vi "CombineVIScreenshots.vi"(6 "Image Types":T1[](array[typedef]), 8 "error in (no error)":errorcluster, 9 "Output Folders":T5, 10 "VI 2 Screenshots in":T2, 11 "VI 1 Screenshots in":T2) -> (0 "error out":errorcluster)   [LabVIEW 2015, in "VIDiff_Screenshots.lvlib"]
uses:
  Screenshots/VIDiff_Screenshots.lvlib
  Utilities/Output Folders.ctl
  Screenshots/VI Screenshots.ctl
  Screenshots/Screenshot Info.ctl
  Screenshots/Screenshot Type.ctl
  Utilities/FilePaths.ctl
  Utilities/VIDiff_Utilities.lvlib
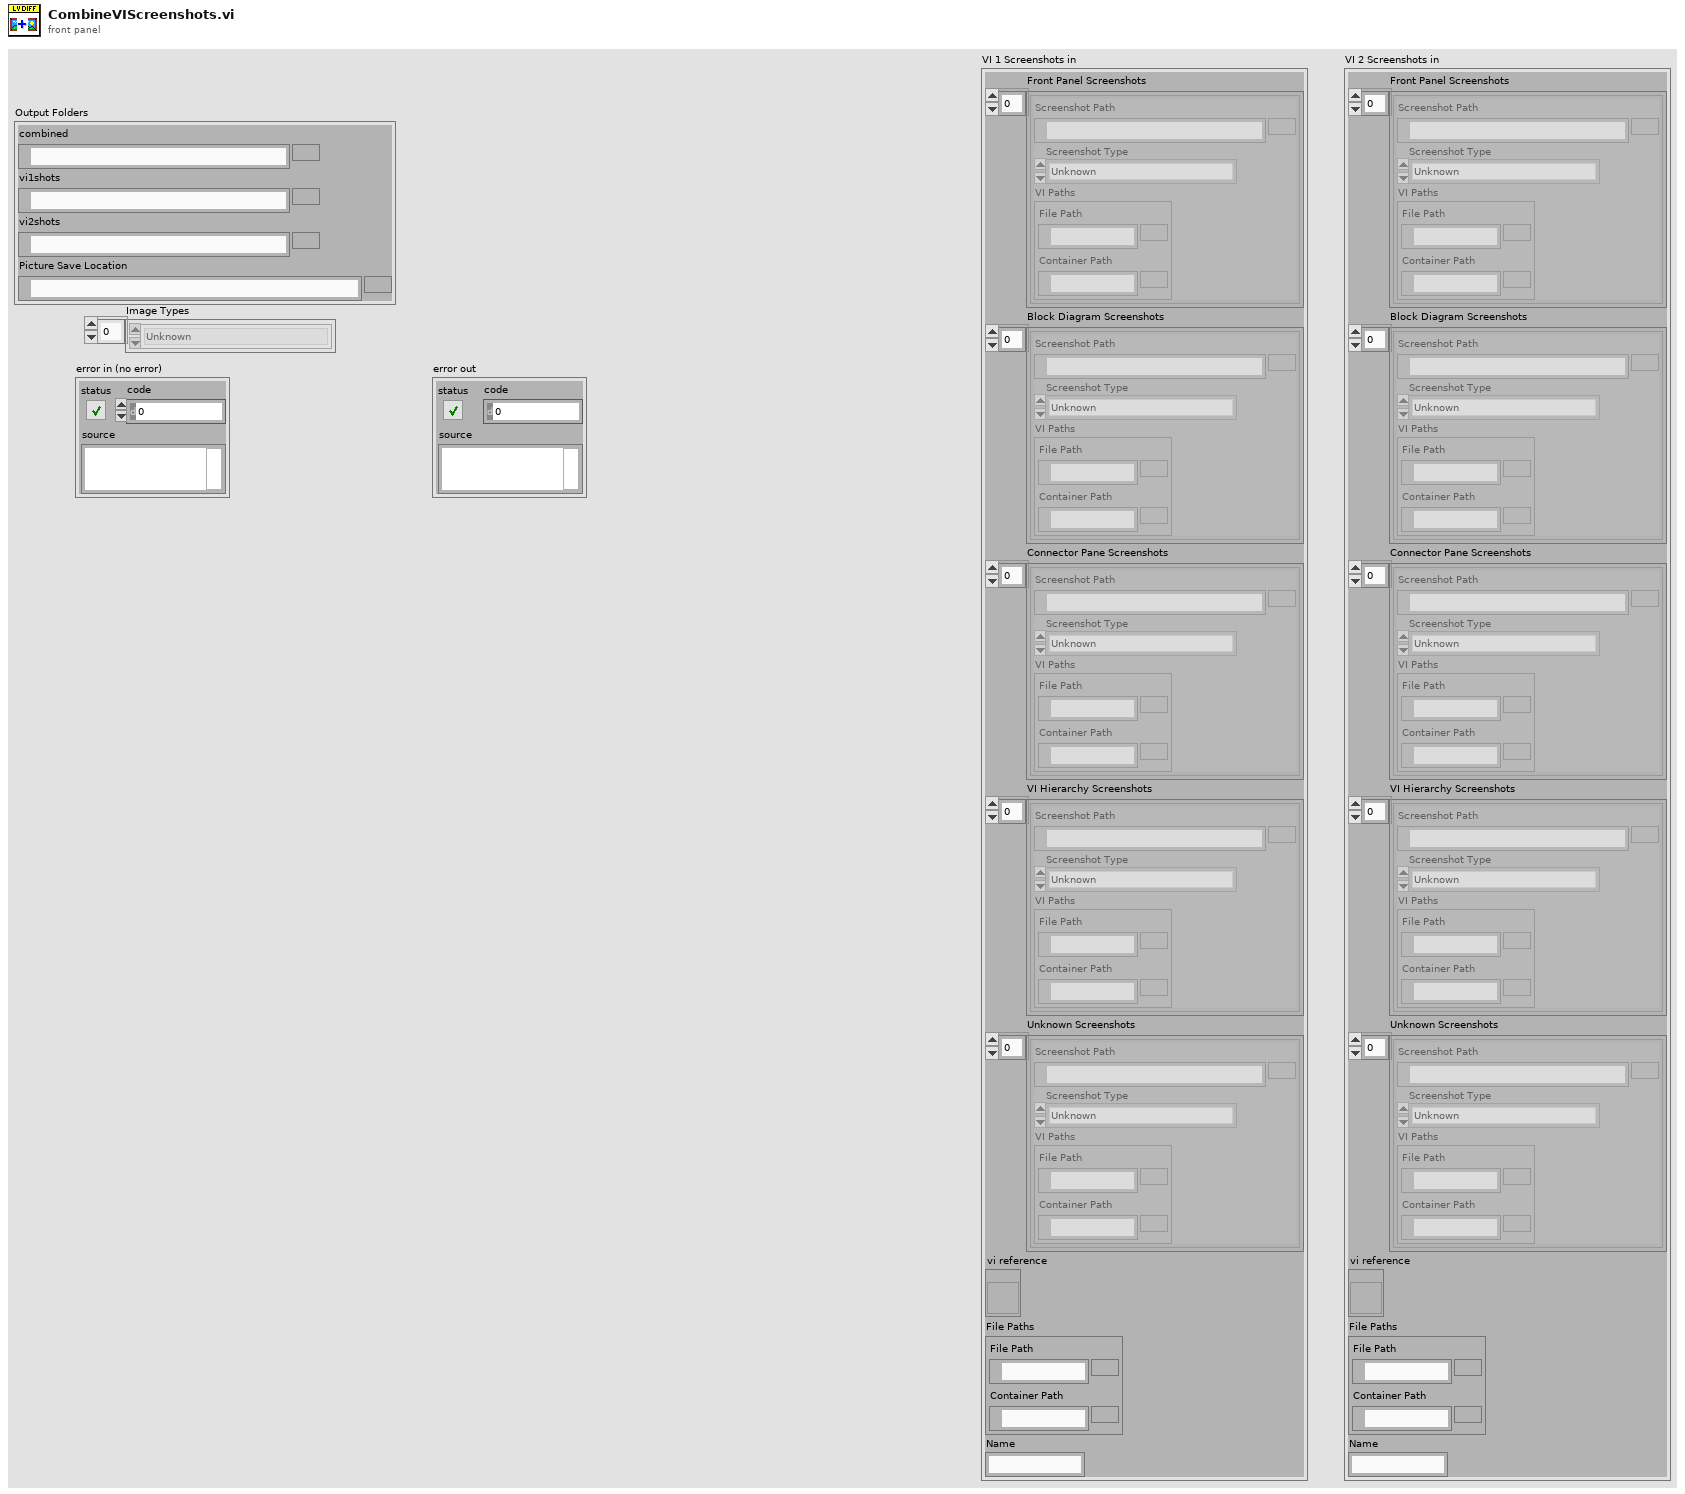
[diagram p1: front panel]
types:
  T1 = typedef "VIDiff_Screenshots.lvlib/Screenshot Type.ctl" = enum16{"Unknown", "Front Panel", "Connector Pane", "Block Diagram", "VI Hierarchy"}
  T2 = typedef "VIDiff_Screenshots.lvlib/VI Screenshots.ctl" = cluster{"Front Panel Screenshots":T3[], "Block Diagram Screenshots":T3[], "Connector Pane Screenshots":T3[], "VI Hierarchy Screenshots":T3[], "Unknown Screenshots":T3[], "vi reference":refnum<vi>, "File Paths":cluster{"File Path":path, "Container Path":path}, "Name":string}
  T3 = typedef "VIDiff_Screenshots.lvlib/Screenshot Info.ctl" = cluster{"Screenshot Path":path, "Screenshot Type":T1, "VI Paths":T4}
  T4 = typedef "VIDiff_Utilities.lvlib/FilePaths.ctl" = cluster{"File Path":path, "Container Path":path}
  T5 = typedef "VIDiff_Utilities.lvlib/Output Folders.ctl" = cluster{"combined":path, "vi1shots":path, "vi2shots":path, "Picture Save Location":path}
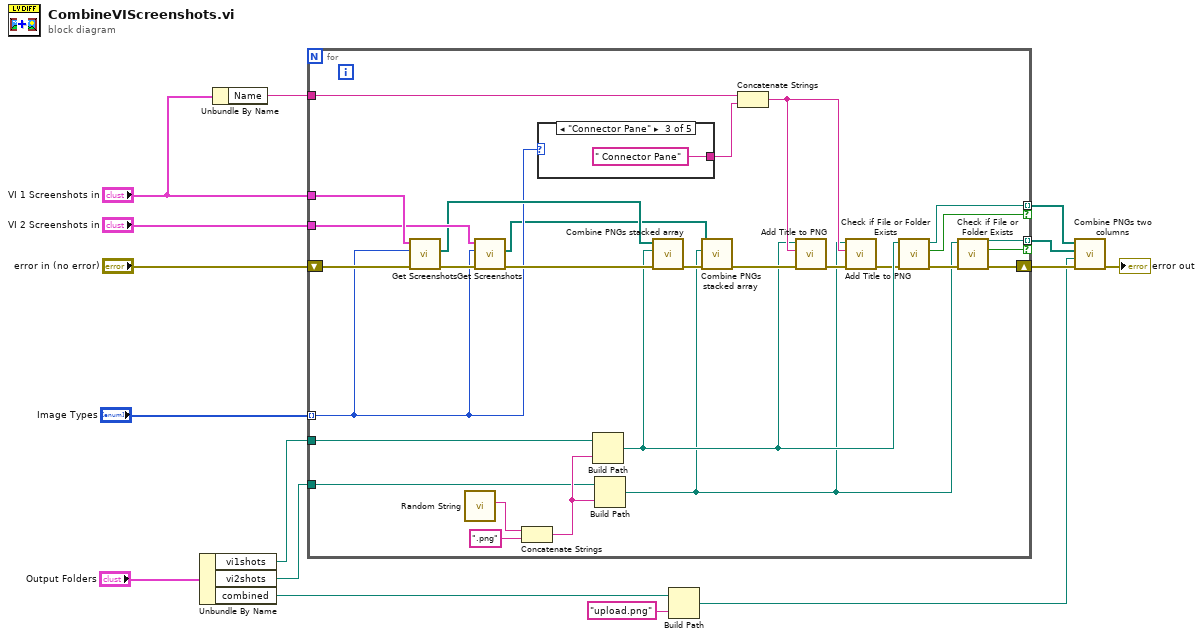
[diagram p0: block diagram]
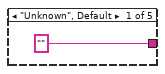
[diagram p2: hidden frame]
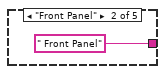
[diagram p3: hidden frame]
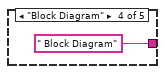
[diagram p4: hidden frame]
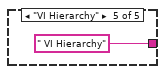
[diagram p5: hidden frame]
diagram:
  n1 = Unbundle By Name("Output Folders") -> ("vi1shots"=w7:path, "vi2shots"=w6:path, "combined"=w4:path)
  n2 = Unbundle By Name("VI 1 Screenshots in") -> ("Name"=w1:string)
  n3 = for {
    shift-right: [w23] -> w11
    shift-left: "error in (no error)" -> [w42]
    tunnel: "Image Types" -> [w35] mode=indexing
    tunnel: "VI 2 Screenshots in" -> [w40]
    tunnel: "VI 1 Screenshots in" -> [w43]
    tunnel: w1 -> [w34]
    tunnel: [w21] -> w12 mode=indexing if=w20
    tunnel: [w19] -> w13 mode=indexing if=w18
    tunnel: w7 -> [w17]
    tunnel: w6 -> [w16]
    n4 = call "Get Screenshots.vi"("error in (no error)"=w42, "Screenshot Type"=w35, "VI Screenshots In"=w43) -> ("error out"=w41:errorcluster, "Screenshot Paths"=w39:path[])  [unwired: 7 in]
    n5 = call "Random String.vi"() -> ("Random String"=w38:string)  [unwired: 11 in]
    n6 = call "Get Screenshots.vi"("error in (no error)"=w41, "Screenshot Type"=w35, "VI Screenshots In"=w40) -> ("error out"=w36:errorcluster, "Screenshot Paths"=w29:path[])  [unwired: 7 in]
    n7 = Concatenate Strings(w38, ".png" ("string")) -> (w30:string)
    n8 = case shown="\"Connector Pane\"" w35 {
      tunnel: ["" " Front Panel" " Connector Pane" " Block Diagram" " VI Hierarchy"] -> w33
      frame "Unknown", Default {
      }
      frame "Front Panel" {
      }
      frame "Connector Pane" {
      }
      frame "Block Diagram" {
      }
      frame "VI Hierarchy" {
      }
    }
    n9 = Build Path(base path=w17, name or relative path=w30) -> (appended path=w26:path)
    n10 = Build Path(base path=w16, name or relative path=w30) -> (appended path=w22:path)
    n11 = call "Combine PNGs stacked array.vi"("error in (no error)"=w36, "Output File"=w26, "Input Files"=w39) -> ("error out"=w32:errorcluster)  [unwired: 8 in]
    n12 = call "Combine PNGs stacked array.vi"("error in (no error)"=w32, "Output File"=w22, "Input Files"=w29) -> ("error out"=w31:errorcluster)  [unwired: 8 in]
    n13 = Concatenate Strings(w34, w33) -> (w28:string)
    n14 = call "Add Title to PNG.vi"("error in (no error)"=w31, "Title String"=w28, "PNG File"=w26) -> ("error out"=w27:errorcluster)  [unwired: 8 in]
    n15 = call "Add Title to PNG.vi"("error in (no error)"=w27, "Title String"=w28, "PNG File"=w22) -> ("error out"=w25:errorcluster)  [unwired: 8 in]
    n16 = call <vilib>:"Check if File or Folder Exists.vi"("error in (no error)"=w25, "path"=w26) -> ("error out"=w24:errorcluster, "file or folder exists?"=w20:bool, "dup path"=w21:path)  [unwired: 7 in]
    n17 = call <vilib>:"Check if File or Folder Exists.vi"("error in (no error)"=w24, "path"=w22) -> ("error out"=w23:errorcluster, "file or folder exists?"=w18:bool, "dup path"=w19:path)  [unwired: 7 in]
  }
  n18 = Build Path(base path=w4, name or relative path="upload.png") -> (appended path=w3:path)
  n19 = call "Combine PNGs two columns.vi"("error in (no error)"=w11, "Output File"=w3, "Right Column"=w13, "Left Column"=w12) -> ("error out"=→"error out":errorcluster)  [unwired: 7 in]
